vi "is invalid.vi"(11 "stream publisher in":refnum<class "subscriber.lvclass">) -> (2 "invalid?":bool, 3 "stream publisher out":refnum<class "subscriber.lvclass">)   [LabVIEW 2013, in "data stream.lvlib" / "subscriber.lvclass"]
uses:
  subscriber.lvclass
  subscriber.lvclass/subscriber.ctl
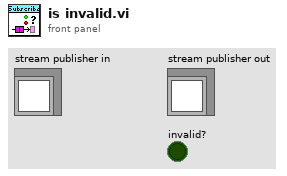
[diagram p1: front panel]
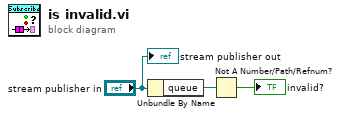
[diagram p0: block diagram]
diagram:
  n1 = Unbundle By Name("stream publisher in") -> ("queue"=w2:refnum<queue>)
  n2 = Not A Number/Path/Refnum?(number/path/refnum=w2) -> (NaN/Path/Refnum?=→"invalid?":bool)
  "stream publisher out" <- "stream publisher in"
